vi "Parse.vi"(8 "Error In":errorcluster, 11 "object in":refnum<class "2024_16.lvclass">) -> (0 "Error Out":errorcluster, 3 "object out":refnum<class "2024_16.lvclass">)   [LabVIEW 2023, in "2024_16.lvclass"]
uses:
  2024_16.lvclass
  Common/AOC_XY(I32).ctl
  2024_16.lvclass/2024_16.ctl
  <vilib>/Utility/error.llb/Trim Whitespace One-Sided.vi
panel:
  out "Map":set{T1}(c389)
  out "Map":bool[][](array[boolean])
  out "Map":cluster{"x":i32, "y":i32}[](array[cluster])
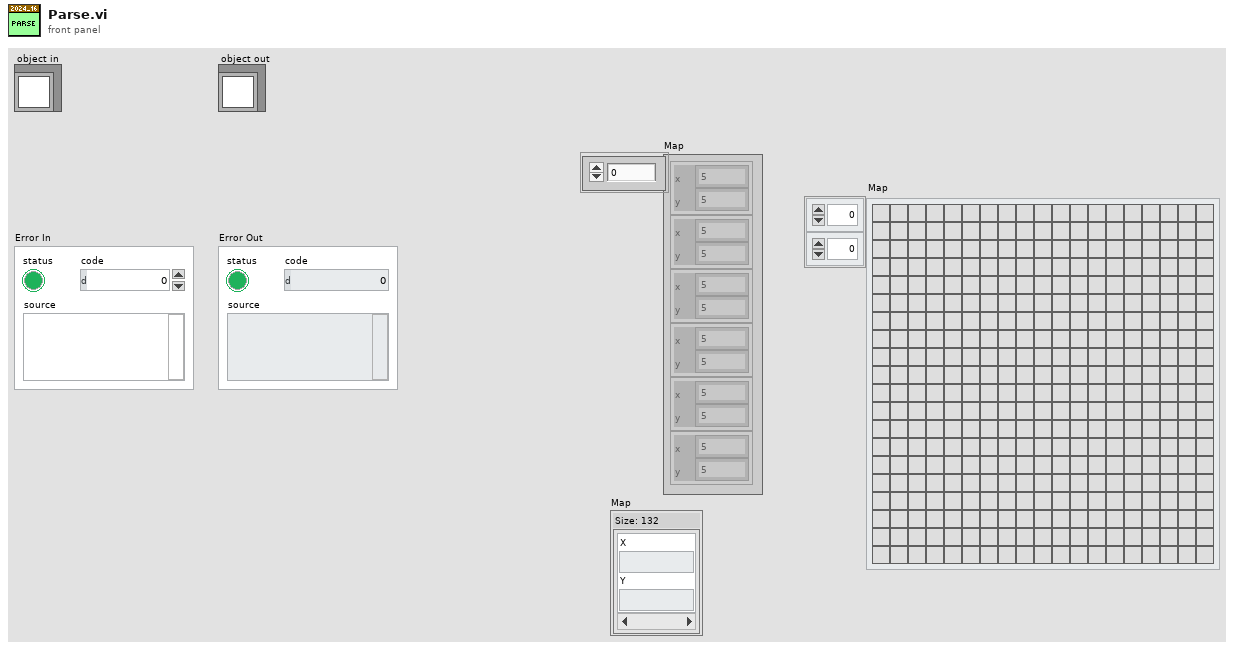
[diagram p1: front panel]
types:
  T1 = typedef "AOC_XY(I32).ctl" = cluster{"X":i32, "Y":i32}
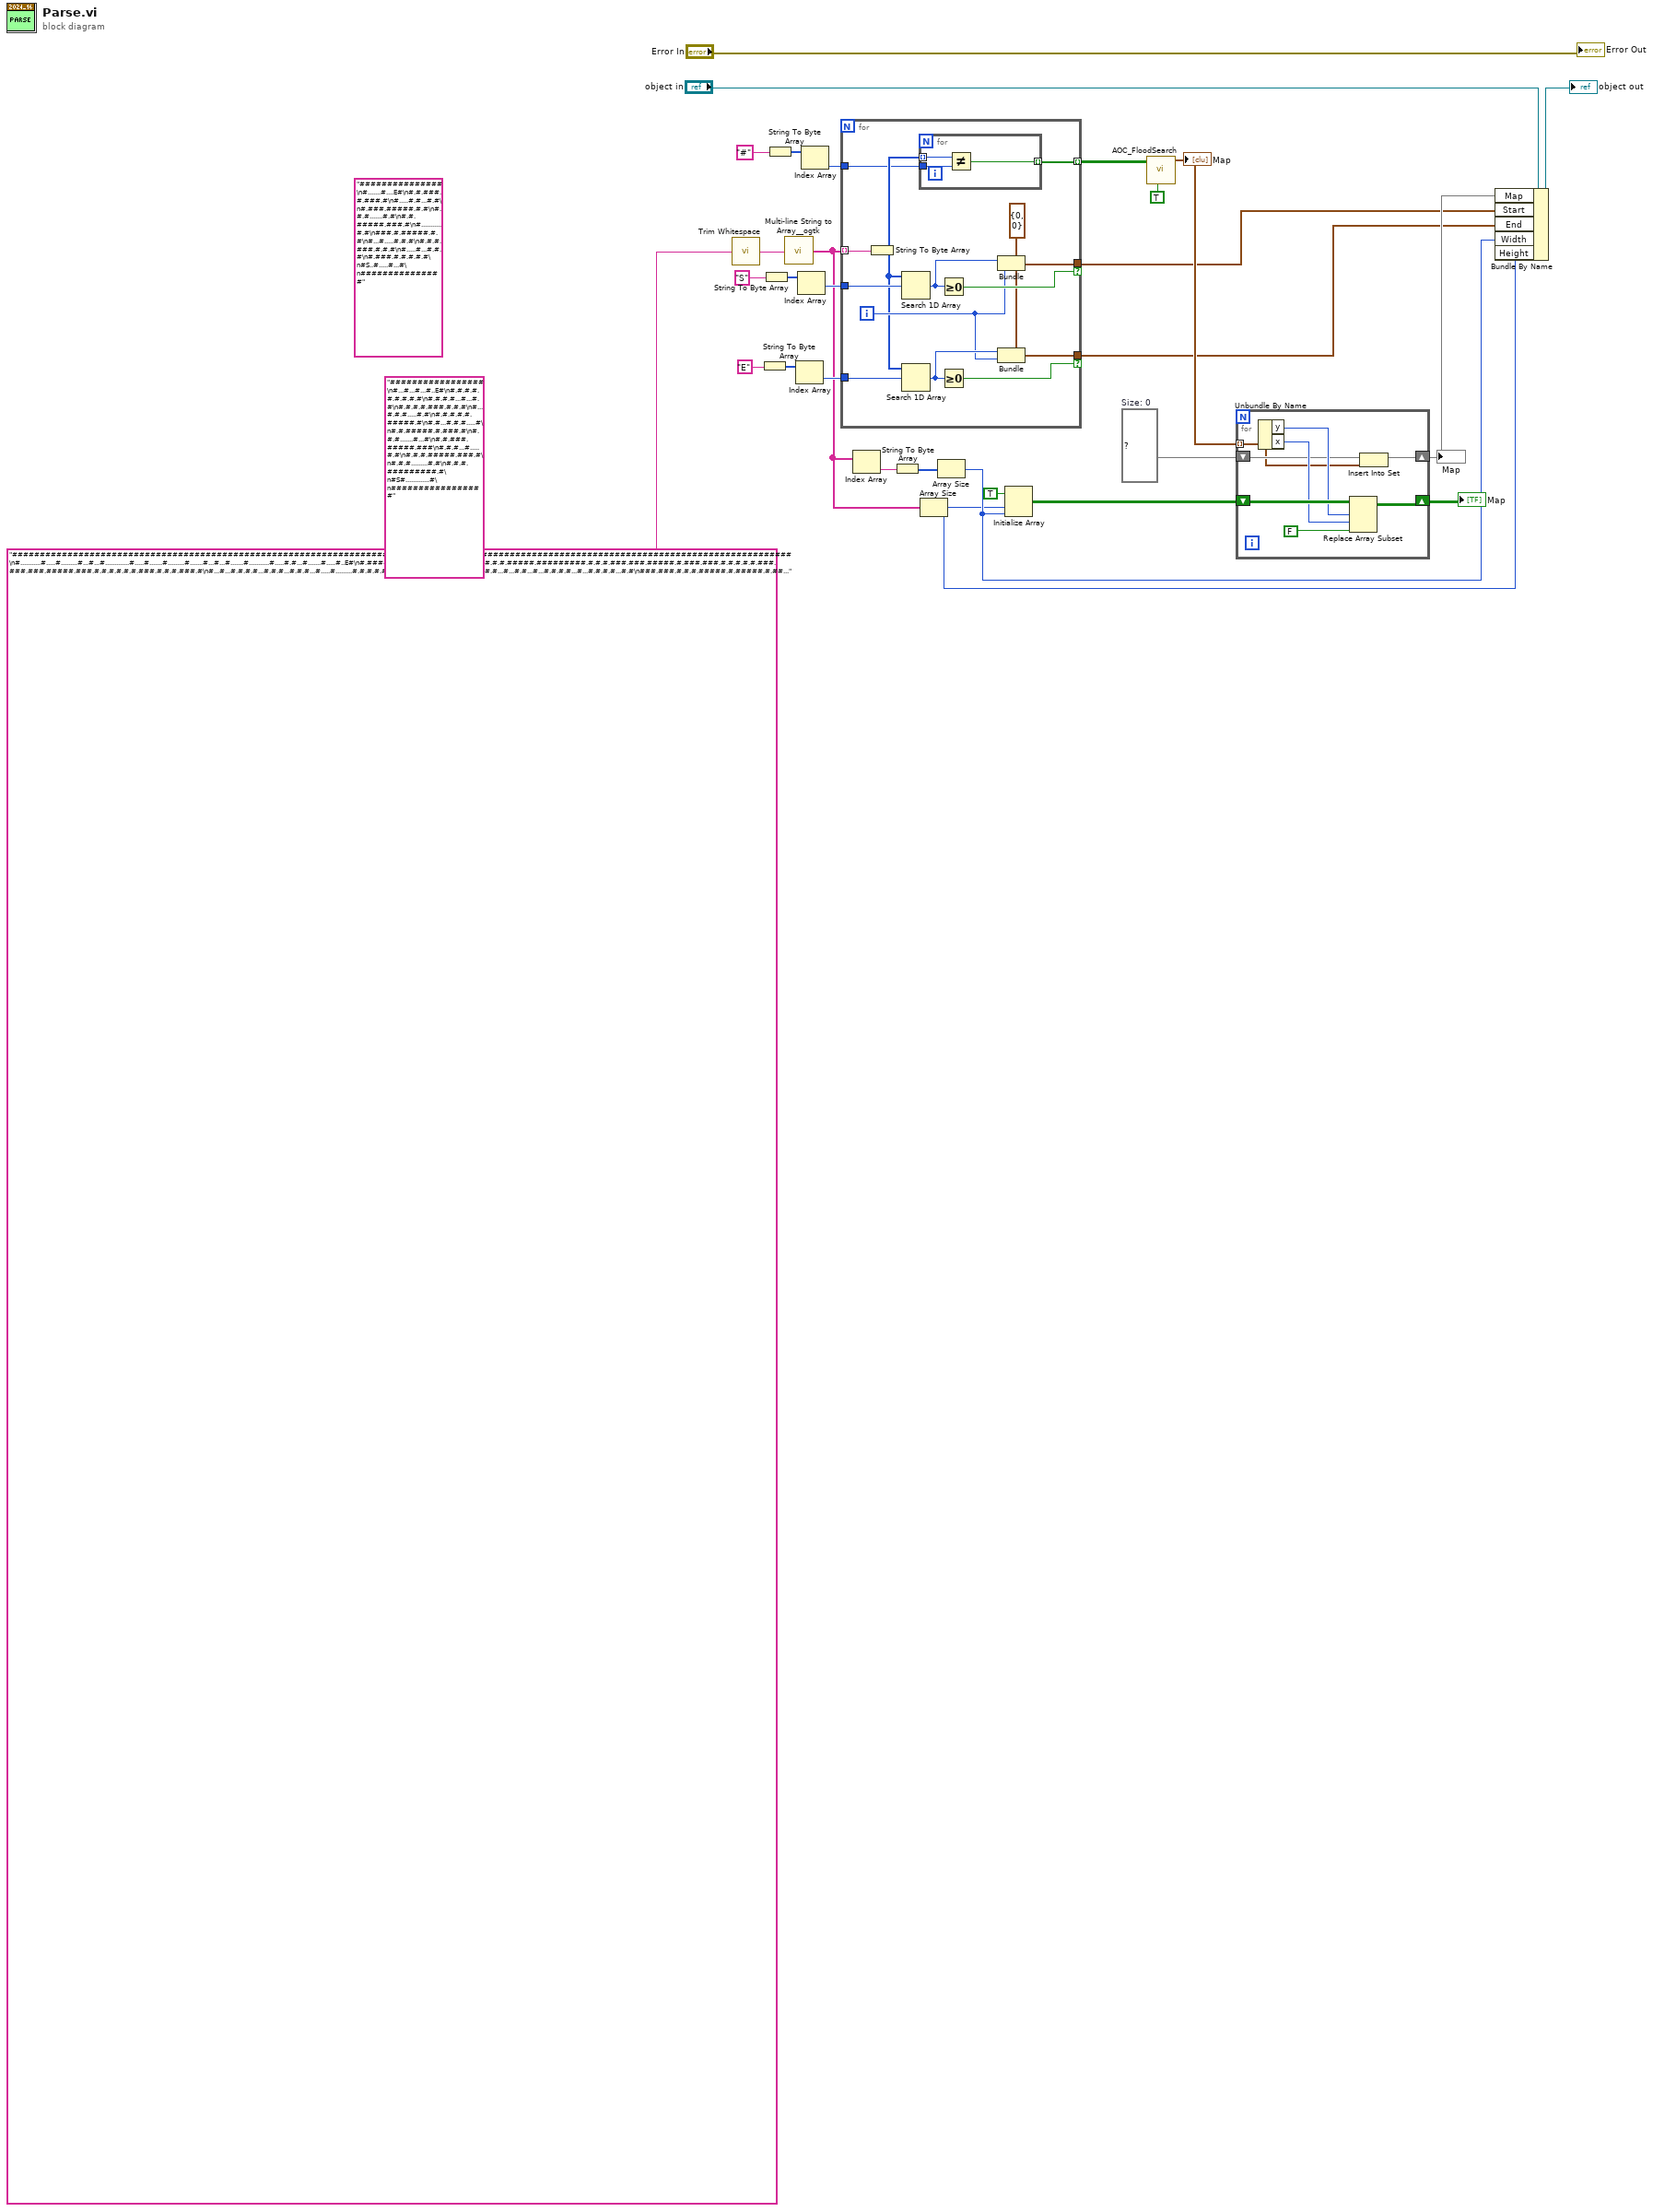
[diagram p0: block diagram]
diagram:
  (unwired) "###############\n#.......#....E#\n#.#.###.#.###.#\n#.....#.#...#.#\n#.###.#####.#.#\n#.#.#.......#.#\n#.#.#####.###.#\n#...........#.#\n###.#.#####.#.#\n#...#.....#.#.#\n#.#.#.###.#.#.#\n#.....#...#.#.#\n#.###.#.#.#.#.#\n#S..#.....#...#\n###############" ("PuzzleInput")
  w8 = set{T1} {}  # Size: 0
  (unwired) "#################\n#...#...#...#..E#\n#.#.#.#.#.#.#.#.#\n#.#.#.#...#...#.#\n#.#.#.#.###.#.#.#\n#...#.#.#.....#.#\n#.#.#.#.#.#####.#\n#.#...#.#.#.....#\n#.#.#####.#.###.#\n#.#.#.......#...#\n#.#.###.#####.###\n#.#.#...#.....#.#\n#.#.#.#####.###.#\n#.#.#.........#.#\n#.#.#.#########.#\n#S#.............#\n#################" ("PuzzleInput")
  n1 = call <vilib>:"Trim Whitespace.vi"("string"="#############################################################################################################################################\n#...........#.....#.........#...#...#.............#.....#.......#.........#.......#...#...#.......#...........#.....#.#...#.......#.....#..E#\n#.#######.#.#.###.#.#.#.#.#.#.#.#.#.#####.#########.#.#.#.###.###.#####.#.###.###.#.#.#.#.#.###.###.###.#####.###.#.#.#.#.#.#.###.#.#.#.###.#\n#...#...#.#.#.#...#.#.#...#.#.#...#.....#.........#.#.#.#.#...#...#.....#...#.#...#.#...#.#...#.#...#...#.#...#...#.#.#.#...#...#.#.#.#...#.#\n###.###.#.#.#.#####.#.#####.#.#########.#.#######.#.#.#.#.#.#.#.###.#######.#.#.###.#.###.###.#.#.###.###.#.###.###.#.#.#######.###.#.###.#.#\n#.#.#...#.#...#...#.#.#...#.#.#.........#...#.....#.#.#.#.#.#.#.#.#.#.....#.#.#.#...#...#.....#.#.#.#...#...#...#...#.#.....#.#.....#.#.#.#.#\n#.#.#.#.#.###.#.#.#.#.#.#.#.#.#.#.###########.#.###.#.#.###.###.#.#.#.###.#.#.#.#.#####.#######.#.#.###.###.###.###.#.#####.#.#######.#.#.#.#\n#.....#.#...#...#.#.#.#.#...#...#.#.......#...#.#...#.#...#.....#.#...#.#.#...#.#.....#...#.....#.#...#...#...#...#...#.....#.......#.#.#.#.#\n###########.#.###.#.#.#.#######.#.###.###.#.#####.###.###.#.#####.#####.#.#####.###.#.###.#.#####.#.#.###.###.#.#.#####.#######.#####.#.#.#.#\n#.....#...#.#...#...#.#...#.....#.....#...#.........#.#...#.......#.....#...#.#...#.#.#...#.......#.#.#...#...#.#.#...#...#...#.#.....#.#.#.#\n#.###.#.#.#.#.#####.#.###.#.#.#.#######.###.#########.#.#########.#.#.#####.#.###.#.#.#.###########.#.#.###.###.#.#.#.###.#.#.#.#.#####.#.#.#\n#...#.#.#.#...#...#.#.#...#.#.....#...#...#...#.....#.#.....#.....#.#...#...#.#...#.#.......#.......#.#...#.......#.#...#...#...#...#...#.#.#\n###.#.#.#.###.#.#.###.#.#######.#.#.#####.#####.###.#.#####.#.#.#######.#.#.#.#.#####.#####.#.#######.###.#####.###.###.#######.###.###.#.#.#\n#...#.#.#...#.#.#.#...#.........#.#...........#.#.#...#...#...#.........#.#...#.......#...#.......#...#.#...#.#.#...#.#.#.......#...#...#...#\n#.###.#.###.###.#.#.#.#########.#.###########.#.#.#######.###.#########.#.#.#.#######.###.#####.#.#.###.###.#.#.#.###.#.#.#######.###.#####.#\n#.....#...#...#.#.#.#.#.....#.....#.......#.....#...........#...#...#.#.#.#.#.......#...#.......#.#.......#.#...#.#...#...#.......#.........#\n#.#.#.###.###.#.#.#.#.#.###.#######.#####.#########.#.#####.###.#.#.#.#.#.#.#######.###.#####.###.###.#####.#.###.#.#.#####.#.#####.#########\n#.#.#...#...#...#.#.#.#...#...#...#.#.#...#...#...#.#.#.....#...#.#...#.#.#...#...#...#.....#...#.....#.....#...#...#.....#.#...........#...#\n#.#.###.###.#.#.#.#.#####.###.#.#.#.#.#.#.#.#.#.#.#.#.###.###.###.#####.#.###.#.#####.#####.#######.###.#####.#########.###.#.#########.#.#.#\n#.............#.#...#...#.#.....#.....#.#.#.#...#.#.#...#.#...#.#.......#...#.#.#.....#...#.......#.#...#.....#...#.....#...#.#.....#...#.#.#\n#.#####.#.###.#.#.#.#.#.#.#.#########.#.###.#####.#####.#.#.###.#.#######.#.#.#.#.#####.#########.#.#.#####.###.#.#.#####.###.#.###.#.###.#.#\n#.....#...#.#.#.#.#...#.#...#.#.....#.......#...#.#.....#.#...#...#.....#.#.#.......#...#.......#.#.#.....#.#...#.#...#...#.#.#.#.#.#.....#.#\n#.###.#####.#.#.###.###.###.#.#.###.#########.#.#.#.#####.###.#.###.###.###.#.#####.#.#.#.#####.#.#######.###.###.#.#.#.###.#.#.#.#.#####.#.#\n#...#.#.......#...#.#...#.....#.#.#...............#.#...#.#...#.#...#.#.....#.#...#...#.#.....#.#.....#...#...#...#.#.#.....#.#.#.#...#.....#\n#####.#.#########.#.#.###.#####.#.#################.#.#.#.#.###.#.#.#.#######.#.#.#########.###.#####.#.###.###.#.#.#.#.#.#.#.#.#.#.#.###.###\n#.....#.....#...#...#.....#.....#.....#.............#.#...#.#.....#.#.........#.#...#.....#.#...#.....#.#...#.#...#...#.#.#...#.#...#...#.#.#\n#.#########.#.#.###.#######.#####.###.#.###.#.###.###.#####.#.#####.#.###.#.#.#.###.#.#.###.#.#.#.#####.#.###.#.###.#.#.#.#####.###.###.#.#.#\n#.....#...#...#...#.......#.#.....#...#...#.....#.#.......#.#.#.....#...#...#.#...#...#...#.......#.......#...#.#.......#...#...#.....#.#.#.#\n#####.#.#.#######.#########.#.#####.###########.#.#########.#.#.#############.###.#######.#.#######.#####.#.###.#.#####.###.#.###.#.###.#.#.#\n#.....#.#.........#...#.....#.#...............#.#.......#...#.#.#...........#...#...#.....#.#.........#...#...#.#.....#.#.....#...#.....#...#\n#.#######.#########.#.#.#####.#############.#.#########.#.###.#.#####.###.#.###.###.#.#####.#.#.#####.#.#####.#.#####.#.#####.#.###.#####.#.#\n#...#...#.....#.....#...#.................#...#.......#.#...#.#.#.....#.............#.......#.#.....#.........#.....#.......#...#...#...#...#\n#.#.#.#.#####.###.#######.###.###########.#.###.#####.#.###.###.#.#####.###.###.#.###.#######.#####.#########.#####.#.#####.###.#.#.#.#.#.###\n#.#...#.....#...#.#.............#...#...#.#.......#.#...#.#.....#.#.........#.#.#.#.....#...#.....#.#.....#...#...#...#.#.....#.#.#...#.....#\n###########.#.#.#.#.###########.#.#.#.#.#.#.###.#.#.###.#.#######.#######.#.#.#.#.#.###.#.#######.#.#.###.#.###.#.#####.#.#####.#.#.#####.#.#\n#...#.....#.#.#...#...#.......#...#...#.#.#.....#.#...#.....#...#.........#.#...#...#.#.#.........#.#...#.#.........#...#...#...#.#.#.#.....#\n#.#.#.###.#.#.###.#.###.#####.###########.###.###.#.#.#####.#.###.#.#.#####.###.#####.#.#######.###.###.#.#.#######.#.#.###.#.###.#.#.#.#.#.#\n#.#...#...#.#.....#...#...#.......#.......#...#...#...........#...#...#...#.......#...#.......#.#.....#.#.#.#...#.....#...#.....#.#.#.#.#...#\n#.#####.###.#.#####.#.#.#.#######.#.#######.###.###.#####.#####.#######.#.#####.#.###.#######.#.#.#.###.#.#.#.#.###########.#####.#.#.#.###.#\n#.#...#.#.....#.....#.#.#...........#.....#.#.....#.....#...#...#...#...#.....#.#...........#.#...#.#...#.#.#.#...........#...#...#...#...#.#\n#.###.#.#####.#.#####.#.###.###.#.#######.#.#####.#.###.###.#.#####.#.###.###.#.#############.#####.#.###.#.#.###########.###.#.#####.###.#.#\n#...#.#...#...#.#...#.#.#.#.....#.#.....#.#.......#...#...#.#...#...#.#.....#.#.............#...#.#.#.#.#.#.#.#.......#.#.#...#.#.......#.#.#\n###.#.#.#.#.#.#.###.#.#.#.#.#######.###.#.#######.###.###.#####.#.###.#.#.#.#.#############.###.#.#.#.#.#.###.###.###.#.#.#.###.#.#######.#.#\n#...#.....#...#...#.#.#...#.#...#...#...#.....#.....#.#.#.......#.#.......#.#.....#...#...#...#.....#.#...#...#...#.....#.#...#...#...#...#.#\n#.#####.#####.###.#.#.#####.#.#.#.###.#####.###.#####.#.#########.#.#####.#####.#.#.#.#.#.#.#.#.#####.#.###.###.#######.#.#.#######.#.#.###.#\n#.....#.....#...#...#.....#.#.#.#...#.#...#.......#...#.......#...#.#...#...#...#...#.#.#.#.#.#.......#.....#.#.......#.#.#.#.....#.#.#...#.#\n#.###.#####.#.###.#.#####.#.#.#.###.#.#.#.#.#######.###.#####.###.#.#.#.###.#.#######.#.#.#.#.#.#.###########.#.#####.###.#.#.###.#.#.###.#.#\n#.#.#.....#.#.....#.#.#...#...#.#...#.#.#.#...#.....#...#...#.#...#...#.#...#...#...#...#.#.#.#...#.#.....#...#.#...#.......#...#...#...#.#.#\n#.#.#####.#.###.###.#.#.#####.#.#.###.#.#.#####.#######.#.#.#.#.#######.#.#.###.###.#####.#.#######.#.###.#.#.#.#.#.#######.###.#######.#.#.#\n#.#...#...#...#...#...#.......#...#.#...#...#...#.......#.#.#.#.......#...#...#...#.#.....#.............#...#.....#...#...#...#...#...#...#.#\n#.###.#.#####.###.###.#####.#.#####.#######.#.#####.#####.#.#.#.#.###.###.#######.#.#.#####.#############.###########.#.#.###.#.#.#.#.#####.#\n#...#.#...#.#.....#...#.#.......#.........#.#...#...#...#.#...#.#...#.....#...#...#...#...#...#.....#...#.#...#.....#.#.#.......#...#...#...#\n###.#.###.#.###.#.#.###.#.#####.###.#.#####.###.#.#####.#.#.#.#.#.#.#######.#.#.#.#.###.#.###.###.#.#.#.#.###.#.###.#.#.#.#####.#####.#.#.###\n#.#...#...#.....#.#...#.#.#...#.....#.#.......#.#...#...#.#...#...#.......#.#...#...#...#...#.....#.#.#.#.....#.#.#.#.#.#.....#.....#.#.#...#\n#.###.#.###.#####.###.#.#.#.#.#####.#.#.###.###.###.#.#.#.###############.#.#########.#####.#######.#.#.#######.#.#.###.#####.#####.###.###.#\n#.....#...#...#.....#.#.#...#.#...#...#.#...#...#...#.#.#.#.....#...#.....#...#...#...#...#.#.......#.#...#...#.#.#...#...#.#...#.#.....#...#\n#.#######.###.###.###.#.#####.#.###.###.#####.###.###.###.#.#.###.#.#.#######.#.#.#.###.###.#.#######.###.#.#.#.#.###.#.#.#.###.#.#######.###\n#...#...#.#.....#.....#...#...#.......#.....#.#...#.......#.#...#.#.#.#...#...#.#.#.#...#...#.#.......#...#.#...#.....#.#.#.....#...#.....#.#\n###.#.#.#.#####.###.###.#.#.#.#.#####.#####.#.#.#.#.#########.#.#.#.#.###.#.###.#.#.#.#.#.#####.#.#.###.###.#####.#######.#.#####.###.#####.#\n#.................#.....#...#.#.....#...#...#...#.#...#.....#.#...#.#.....#.#...#...#.#.#.......#.#...#...#.#...#.......#.#.....#...#.#.....#\n#.#.#.#######.###.###.#######.#####.###.#.#######.###.#.###.#.#####.#.#.#.#.#.#######.###########.###.#.#.#.#.#.#######.#.#####.###.#.###.#.#\n#.#...#.....#.#...#...#.....#.#...#...#.#...........#...#.#.#...#.#.....#.#.#...#...#...........#...#...#...#.#...#...#.#.....#...#.#.....#.#\n#.#.#.#.###.#.#.#######.###.#.#.#.###.#.#####.#####.#####.#.###.#.#####.#.#.###.#.#.#.#####.###.###.#.#.#####.###.###.#.#####.###.#.#######.#\n#...#...#.#.#.#...#.....#.....#.#.....#.....#.....#.......#...#.#.....#...#...#.#.#.#.#...#...#...#.#.#.#...#...#.....#.......#.#.#.......#.#\n#####.###.#.#.###.#.#############.#####.###.#####.#.#########.#.#.#.#.#.#####.#.#.###.#.#.###.###.#.#.#.#.#.#.#.#.#############.#.#.#.###.#.#\n#...#...#.....#...#.......#.....#.........#.....#.#.#.........#...#.#.#.#.....#.#.....#.#...#...#.#.#.#.#.#...#.#.#.....#.......#.#.#...#.#.#\n#.#.#.#.#######.###.#####.###.#.#.#####.###.#####.#.#.###.#######.#.#.###.#####.#.#####.###.###.###.#.#.#####.#.###.###.#.#.#####.#.###.###.#\n#.#...#.....#...#.......#.#...#.#.....#.#...#.......#.#...........#.#.....#...#.#.#.....#.#...#.#...#.#.....#.#...#...#...#.......#.........#\n#.###.#####.#.###########.#.###.#####.###.###.#####.#.#.###########.#####.#.#.#.#.#.#.#.#.###.#.#.#########.#.###.###.#############.#.#.#####\n#.#.........#.#...........#.#...#...#...#...#.......#.#.....#...#...#.....#.#...#.#...#.#...#...#.#.......#.#...#.#...#.....#...........#...#\n#.###.#####.#.###.#########.#.###.#####.###.#####.###.#####.#.###.###.###.#.#####.#.#.#.###.#.###.#.#.###.#.###.#.#.#####.#.###########.#.#.#\n#.........#.#.#...#.........#...#...........#.....#...#.....#.#...#...#.#.#.......#.#.#.......#...#.#...#.#.#.#.#.#.#.....#.......#.....#.#.#\n#####.###.#.#.#.#####.#.#######.#############.#.###.###.#####.#.###.###.###.#.#####.#.#.#.#####.###.###.#.#.#.#.#.#.#.###########.#####.#.#.#\n#.........#.#...#...#.#.#.....#.#...#.....#...#.#...#.#.......#.#.....#...#.#...#...#...#.......#...#...#...#.#.#...#.......#.....#.....#.#.#\n#.###.#####.#####.#.#.#.###.###.#.#.#.###.#.#.###.###.#####.#.#.#.#######.#.###.#.#.###############.#.#######.#.#####.#####.###.###.###.#.#.#\n#.......#.........#.#.#...#...#...#...#.....#.....#...........#.#...#...#...#...#...#.............#.#.#.....#...#.....#...#...#.....#.#.#...#\n#.###.#.#.#.#.#####.###.#.#.#.#########.#######.###.###########.###.#.#.#####.#####.#.#######.#.#.###.#.###.#.###.#####.#.###.#######.#.#.#.#\n#.#...#.#...#...#.....#.#.#.#...#.....#.#.......#...#...........#.....#.....#.....#.#.#.....#...#.....#...#.#.#.........#...#...#.........#.#\n#.#.#.#.###.###.#####.#.#.#.###.#.#.###.#.#######.###.#####.#.###.#########.#####.#.#.#.###.#.#############.#.#########.#######.#######.###.#\n#...#.#.............#.#.#.#.......#.....#.#.........#.#.#...#.......#.......#...#.#.#.#...#...#.........#...#.......#...#.....#...#.....#...#\n###.###.#.#.#.#####.#.###.###.###.#######.###########.#.#.###########.#####.#.###.#.#.#.#.#.###.#######.#.#.###.###.###.#.###.#.#.#.#.#.#.#.#\n#.....#.#.#.....#...#.....#...#.....#.....#...........#.#.#...........#...#.#.#...#.#...#.#...#.......#...#.#.....#...#.#.#.....#.....#...#.#\n#.###.###.#####.#.###.#####.#.#.#####.#.###.###########.#.###.#########.###.#.#.#.#.###.#.###.#######.#####.#.###.###.#.#.#.#####.###.#.#.#.#\n#...#...#.....#.#...#.#...#.#.#...#.......#.#...........#...#.........#.....#.#.#...................#.#...#...#...#...#...#.....#.#.......#.#\n#.#.###.#.###.#.###.###.#.#.#####.#.###.#.#.#.#######.#.###.#.#.#.###.#.#####.#.#.#########.#######.#.#.#.###.#.###.#.###.#.###.###.#.###.#.#\n#.#.#...#.#...#.#.#.#.....#.....#.#.....#...#.#.........#.#...#.#.#.#.#.......#.#.#.............#.#.#.#.#.......#...#...#...#.#.....#.....#.#\n#.#.#.###.#.###.#.#.#.###.#####.#.###########.#.#.###.###.#######.#.#.#######.#.#.#.###.#######.#.#.#.#.###########.###.###.#.#######.#.#.#.#\n#.#.#...#...#.#.#.#.#...#.....#.........#.....#.#...............#.#...#.......#.#.#.#.#...#...#...#...#.......#.....#.#.....#.#.........#.#.#\n#.#.###.###.#.#.#.#.###.#####.#########.#.#####.###.###########.#.#####.#######.###.#.###.#.#.###.#.#.#######.#.###.#.#.#####.#.###.#.#.#.#.#\n#.#...#.....#.#...#...#.....#.#...#...#...#.....#...#...#...#.....#...#.#...#.#.....#...#.#.#.#...#.#.....#.#...#...#...#...#...#.#.....#.#.#\n#####.#######.#.#.#.#.#####.#.#.#.###.###.#.###.#.#.#.#.#.#.#####.#.#.#.#.#.#.#######.#.#.#.#.#####.#.###.#.#####.###.###.#.#.###.###.#.#.#.#\n#...#.......#.#...#.#.#...#.#...#...#.....#.#.....#...#...#...#...#.....#.#.....#.....#...#.#...#...#.#.#.#...#...#.......#...#.......#...#.#\n#.#.###.###.#.#.###.###.#.#.#######.#.#.#.#.###.###########.#.#.#.#.#####.#######.#########.###.#.###.#.#.###.#.#####.#.###.###.###.#.#.#.#.#\n#.#.#.......#.#...#.....#.......#...#.#...#.#...#.........#.#.#.#...#.#.........#.....#...#.#.#...#.....#...#...#...#.........#...#.#...#.#.#\n#.#.#.#.#####.#.#########.#######.#########.#.###.#######.###.#.#.###.#.#######.#####.#.#.#.#.#####.#######.#.###.#.#########.#####.#.#.#.#.#\n#.#...#...#.....#.......#.#.#.....#...#.....#.#...#...........#.#.#.............#.....#.#...#.......#.......#.....#.........#.#.....#.#...#.#\n#.#####.#.#####.#.#####.#.#.#.#####.#.#.#####.#.###############.#.#########.###.#.#####.#####.#######.#####################.#.#.#####.###.#.#\n#.#...#.#.#...#.#.#.....#.#.#.#.....#.#.#...#.#.........#.......#.......#...#.#.#.....#.....#.#.....#.......#...............#...#...#.#.#...#\n#.#.#.#.#.#.#.###.#.#####.#.#.#.#####.#.#.#.#.#########.###############.#.###.#.###.#.#.###.#.#.###.#######.#.#######.###########.#.#.#.#.#.#\n#.#.#...#...#.#...#.#...#...#...#...#...................#.............#...........#.#.#...#.#...#...#.....#.#.......#.#...#.....#.#.#.#...#.#\n#.#.###.#####.#.###.#.#.###.#####.#.#############.###.###.#####.###########.#####.#.#.#.#.#.#####.###.#.#.#.#.#####.#.###.#.#.#.#.#.#.###.#.#\n#.......#...#...#.#...#.#.....#...#.#.......#...#...........#...#.........#.#...#...#...#...#...#...#.#...#...#.....#...#...#.#...#...#...#.#\n#.###.#.#.#######.#####.#######.###.#.#####.#.#.#############.###.###.###.#.#.#.###.#########.#.###.#.#.#####.#.#.#####.#####.###.#####.#.#.#\n#.#...#.#.....#.......#...#.......#.#.....#...#.#.....#.....#...#.#.....#...#.#.......#...#...#.....#.#.......#.#.....#.......#...#.....#.#.#\n#.#.###.#.###.#.#.#######.#.###.###.#####.#####.#.###.#.###.###.#.###.#.#####.#####.#.###.#.#################.#.###.#.#########.###.#####.#.#\n#.....#.#.....#.#...#.....#.........#...#.#...#...#.#.#...#...#.#...#.#...#...#.#.......#.#.#.............#...#.....#.....#.........#...#...#\n#####.#.#.#####.###.#.###.#.#.#######.#.#.#.#.###.#.#.###.###.#.###.#.#.#.#.###.#.#####.#.#.#.###.#.#####.#.#.###########.#.#####.#.#.#.#.###\n#.#.....#.....#.#...#.#...#.#.........#.#.#.#.......#...#.#.#.#.#...#.#.#.#.#...#.#.....#.#.#.#...#...#...#.#...........#.#...#.#.#...#.....#\n#.#.###.#.#.#.#.#.#.#.#####.###########.#.#.###.#######.#.#.#.#.#.###.#.#.#.###.#.#####.#.#.###.#.#.###.###.#####.#.###.#.###.#.#.#.#.###.#.#\n#.#.#.....#.#...#.#.#.#...#.......#...#...#...#.......#.#.#.....#...#...#.#.#...#.....#...#.#...#.#.....#.......#.#...#.....#...#.#...#...#.#\n#.#.#.#.#.#####.#.###.#.#.#######.#.#.#######.#######.#.#.#####.###.###.#.#.#.#.#####.#.###.#.###.#.#####.#####.###.#.#.###.#####.#.###.#.###\n#.#...#.#.....#.#.#...#.....#.......#...#...........#.#.#.....#...#...#.#.#...#.......#.#...#...#.#...#.#.#.....#.....#...#...#...#...#.#...#\n#.#####.#.###.###.#.###.###.#.#########.#######.#####.#.#####.#.#####.###.###.#####.#.###.#.#.#.#.###.#.#.#.###.#.###.#######.#.###.#.#.#.#.#\n#...#...#.........#.......#.....#.....#.....#...#...#.#...#...#.#.....#...#...#...#.#...#...#.#.#...#.#...#...#.#.#.#.#.....#.#.....#.#.#.#.#\n#.###.#.#.#######.###########.###.###.#####.#####.#.#.###.#.#####.#####.###.###.#.#####.###.###.#.#.#.#.#####.#.#.#.#.#.###.#.#####.#.#.#.#.#\n#...#.#...#...#.......#...#.....#.#...#...#.#.....#.....#.#.#...#.#.....#...#...#.........#.....#.#...#...#.#.#.#.#.#.#.#...#...............#\n#.#.#.#.#.#.#.#########.#.#.###.#.###.###.#.#.###.#######.#.#.#.#.###.###.###.###########.#######.#######.#.#.#.#.#.#.#.#.#.#.#.#.#.#####.#.#\n#.#.#.#...#.#...........#...#...#...#...#.....#...#.......#...#.....#.#...#.#...#.....#...#.....#...#...#.#.#.#.#.#.#...#.#...#.#.#.....#.#.#\n#.#.#.#.###.#####.###########.#####.###.#.#########.#######.#######.#.#.###.###.#.#.#.#.###.###.###.#.#.#.#.#.###.#.#####.#.###.#.#.###.#.#.#\n#.#.#.#.#.........#.................#.#.#...........#.#.....#.....#...#...#...#.#...#...#...#...#...#.#.#...#...#.#.....#.#.#...#.....#.#.#.#\n#.#.#.#.#.###.#####.#.###.#########.#.#.#####.#######.#.#####.###.#######.###.#.#.#.#####.###.###.###.#.###.###.#.#####.#.#.###.###.#.#.#.#.#\n#.#...#.#...#.#.....#...#...#.......#.........#.....#.#...#...#.#.....#.............#.#.....#...#...#.#...#.#.#.#.#.....#.#...#.......#.#...#\n#.#####.###.#.#.#######.#####.#####.#.###########.#.#.###.#.###.#####.#.#####.###.#.#.#.###.###.###.#.###.#.#.#.#.#.#.#.#.###.#####.#.#.#.#.#\n#.#.....#...#.#...#.....#.....#...#.#.#...#.......#.#...#.......#...#.#.#...#...#.#.#.#.#...#.....#...#.#.#...#.....#.#.....#.......#.#...#.#\n#.#.#####.#######.#.###.#.###.#.###.###.#.###.#####.#.###.#####.#.###.#.#.#.#####.#.#.#.#.#.#.###.#####.#.###.#######.#.###.#######.#######.#\n#...#...#.#.......#...#.#.#.....#...#...#...#.#.....#.#...#.....#...#...#.#.......#...#...#.#.#...#.....#.#.#.#.#.......#.........#.........#\n#.###.#.#.#.#########.###.#.#.#.#.###.#####.#.#####.#.#.#.#.#.#####.#####.#######.#########.#.#.#####.###.#.#.#.#.#.###.#.#######.###########\n#.#...#...#...#.....#...#.#.#...#.....#.....#.....#...#...#.#...#...#...#.#...#...#.................#...#.#.....#.#...#.#.#...#...#.........#\n#.#.#.#.#####.#.#.#####.#.#.#.#########.#######.#.#######.#.#.#.#.#.#.###.###.#.###.#.#####.#.#.#.#.###.#.#####.#.###.#.#.#.#.#####.#####.#.#\n#.#.#.#.#...#.#.#.....#...#.#.#...#...#...#...#.#.#.......#.#.#...#.#...#...#...#...#.......#.#...#.....#...#...#.#...#.#.#.#.....#...#...#.#\n###.#.#.#.#.#.#.#####.#####.#.#.#.#.#####.#.#.#.#.#.#######.#.#####.###.###.###.#.###########.#########.###.#.###.#.###.###.#####.#.#.#.###.#\n#...........#.#...#...#.....#...#...#.....#.#.#.#.....#...#...#...#.......#...#.#...#.#.....#.......#.....#.#...#.......#.......#...#.#.#...#\n#.###.###.#.#.###.#.#.#.#####.#####.#.#####.#.###.#####.#.###.#.#########.###.#####.#.#.#.#########.#######.###.#.#######.#######.###.#.#####\n#.#.....#.#...#.....#...#...#.......#.......#...#.#.....#.....#.#.........#...#.....#.#.#.....#.#...#.......#...#...........#...#...#.#.....#\n#.###.###.#####.#########.###.#################.###.#####.#.#.#.#.#########.###.#####.#.###.#.#.#.###.#######.###############.#.###.#.#####.#\n#.........#...#.#...#.........#...#.................#.....#.#...#.#.....#...#...#...#...#.#.#...#.....#.....#...........#.....#...#...#.....#\n#.###.#####.#.#.#.#.#.#####.#.#.#.#.#.#########.#.###.#.#.#.#####.###.#.#.###.###.###.###.#.###.#######.#.###.###########.#######.#####.###.#\n#.#.........#...#.#.#.#.......#.#...#.#...#...#.#...#.#.#.#.#.....#...#.#...#.#...........#.#...#.....#.#.....#...#...#...#.#...#...#...#.#.#\n#.###.###########.#.#.###.###.#.#######.#.#.#.#####.###.#.#.#.#####.###.###.#.#############.#.###.###.#########.#.#.#.#.###.#.#.###.#.###.#.#\n#S....#...........#.......#...#.........#...#...........#.#.........#.....#.................#.....#.............#...#...#.....#.......#.....#\n#############################################################################################################################################" ("PuzzleInput")) -> ("trimmed string"=w26:string)  [unwired: 1 in]
  n2 = String To Byte Array(string="E") -> (unsigned byte array=w23:u8[])
  n3 = String To Byte Array(string="S") -> (unsigned byte array=w24:u8[])
  n4 = String To Byte Array(string="#") -> (unsigned byte array=w19:u8[])
  n5 = call <userlib>:"Multi-line String to Array__ogtk.vi"("string"=w26) -> ("lines"=w13:string[])
  n6 = Index Array(array=w23) -> (element=w20:u8)  [unwired: 1 in]
  n7 = Index Array(array=w24) -> (element=w21:u8)  [unwired: 1 in]
  n8 = Index Array(array=w19) -> (element=w17:u8)  [unwired: 1 in]
  n9 = for {
    tunnel: w13 -> [w43] mode=indexing
    tunnel: w21 -> [w42]
    tunnel: [w40] -> w5 if=w39
    tunnel: w20 -> [w36]
    tunnel: [w34] -> w4 if=w33
    tunnel: w17 -> [w31]
    tunnel: [w30] -> w15 mode=indexing
    i -> [w35]
    w37 = T1 {"X"=0, "Y"=0} ("XY")
    n10 = String To Byte Array(string=w43) -> (unsigned byte array=w32:u8[])
    n11 = Search 1D Array(1D array=w32, element=w42) -> (index of element=w41:i32)  [unwired: 1 in]
    n12 = Search 1D Array(1D array=w32, element=w36) -> (index of element=w38:i32)  [unwired: 1 in]
    n13 = for {
      tunnel: w32 -> [w46] mode=indexing
      tunnel: w31 -> [w45]
      tunnel: [w44] -> w30 mode=indexing
      n14 = Not Equal?(x=w46, y=w45) -> (x != y?=w44:bool)
    }
    n15 = Greater Or Equal To 0?(x=w41) -> (x >= 0?=w39:bool)
    n16 = Greater Or Equal To 0?(x=w38) -> (x >= 0?=w33:bool)
    n17 = Bundle(cluster=w37, "X"=w41, "Y"=w35) -> (w40:T1)
    n18 = Bundle(cluster=w37, "X"=w38, "Y"=w35) -> (w34:T1)
  }
  n19 = Index Array(array=w13) -> (element=w14:string)  [unwired: 1 in]
  n20 = String To Byte Array(string=w14) -> (unsigned byte array=w12:u8[])
  n21 = Array Size(array=w13) -> (size(s)=w2:i32)
  n22 = Array Size(array=w12) -> (size(s)=w3:i32)
  n23 = Initialize Array(TRUE ("4 (T) or 8 (F)"), w2, w3) -> (w10:bool[][])
  n24 = call "AOC_FloodSearch.vi"("4 (T) or 8 (F)"=TRUE, "DataIn"=w15) -> ("PixelsFound"=w9:cluster{"x":i32, "y":i32}[])  [unwired: 6 in, 3 out]
  "Map" <- w9
  n25 = for {
    tunnel: w9 -> [w48] mode=indexing
    shift-right: [w50] -> w7
    shift-left: w10 -> [w54]
    shift-right: [w47] -> w6
    shift-left: w8 -> [w49]
    n26 = Unbundle By Name(w48) -> ("y"=w52:i32, "x"=w53:i32)
    n27 = Replace Array Subset(array=w54, new element=FALSE, index (row)=w52, index (col)=w53) -> (w50:bool[][])
    n28 = Insert Into Set(10:w48, 11:w49) -> (3:w47:set{T1})  [unwired: 1 out]
  }
  "Map" <- w7
  "Map" <- w6
  n29 = Bundle By Name(cluster="object in", "Map"=w6, "Start"=w5, "End"=w4, "Width"=w3, "Height"=w2) -> (→"object out":refnum<class "2024_16.lvclass">)
  "Error Out" <- "Error In"
